vi "Read_Write_ADAM_setup.vi"(3 "Mode":T1(ring)) -> ()   [LabVIEW 2012]
uses:
  ADAM Client/Sub VIs/ADAM Controls/Channel_State.ctl
  Anemometry/Anemometry Sub Vis/Globals/Constants_global.vi
  Anemometry/Anemometry Sub Vis/Globals/Gas_management_global.vi
  Exp conditions/EnFlo_Tun_Setup_global.vi
  ADAM_Global.vi
  Channel_Description_Global.vi
panel:
  out "Setup Filename":string
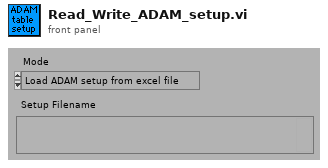
[diagram p1: front panel]
types:
  T1 = enum16{"Load ADAM setup from excel file", "Save ADAM setup to excel file"}
  T2 = typedef "Channel_State.ctl" = enum16{"On", "Off", "Always On", "Always Off"}
  T3 = typedef "Ch_description_ADAM.ctl" = cluster{"Ch Name":string, "Type":T4, "Function":T5, "Ch State":T2, "Calibration type":T6, "A":dbl, "B":dbl, "C":dbl, "D":dbl, "Comments":string, "Address":T7, "String":string, "Duty":u16}
  T4 = typedef "Module_type_ADAM.ctl" = string
  T5 = typedef "Function_ADAM.ctl" = enum16{"Analogue Input", "Digital Input", "Event counter", "Event rate", "Analogue Output", "Digital Output", "Relay Output"}
  T6 = typedef "Calib_type_ADAM.ctl" = enum16{"Raw", "Bx + A", "Cx^2 + Bx + A", "Dx^3 + Cx^2 + Bx + A", "In Band", "Hi-Tec Q", "Hi-Tec M_dot", "Text"}
  T7 = typedef "Address.ctl" = cluster{"Main":i32, "Ch.":i32, "Sub":i32, "Port Name":string}
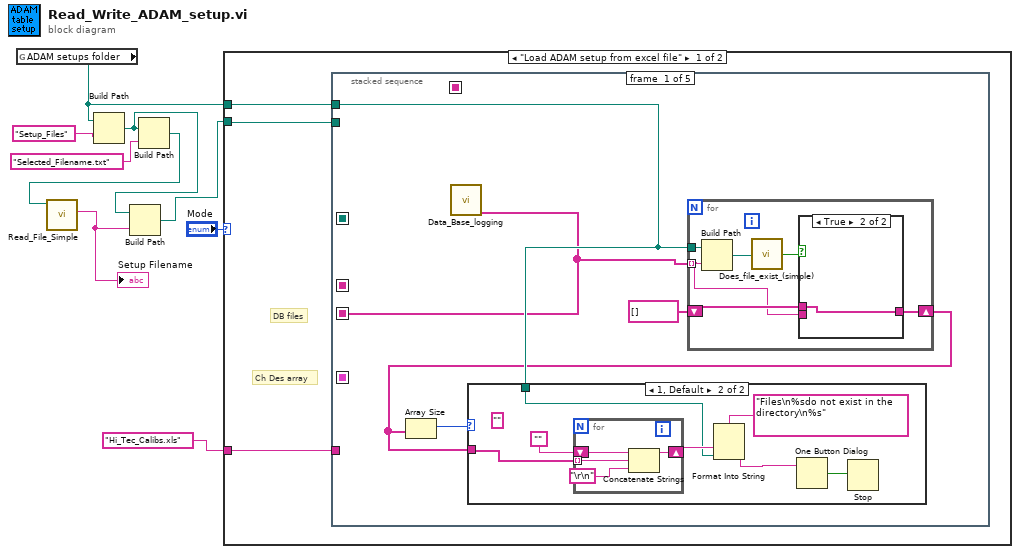
[diagram p0: block diagram]
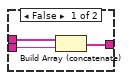
[diagram p3: hidden frame]
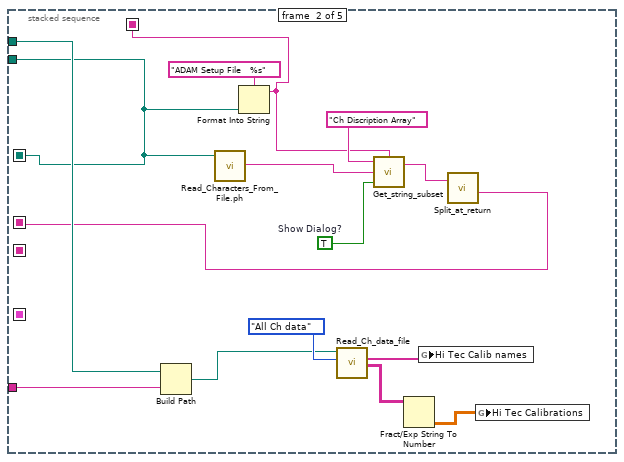
[diagram p4: hidden frame]
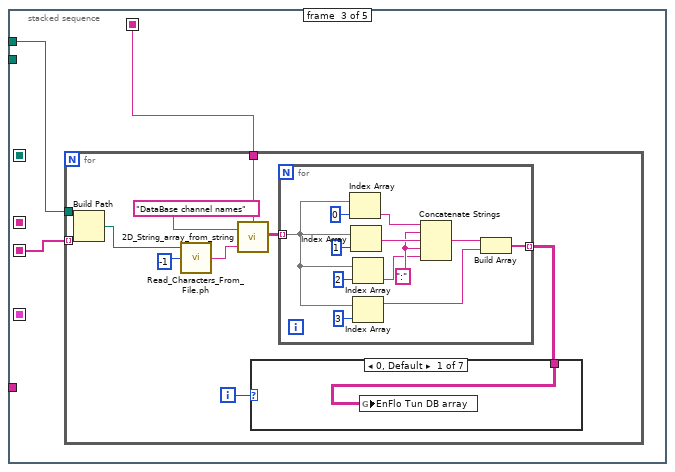
[diagram p5: hidden frame]
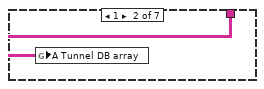
[diagram p6: hidden frame]
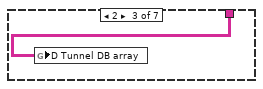
[diagram p7: hidden frame]
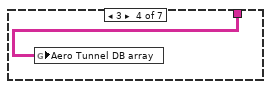
[diagram p8: hidden frame]
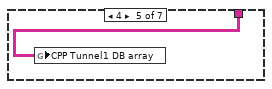
[diagram p9: hidden frame]
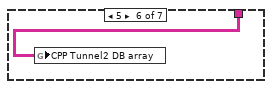
[diagram p10: hidden frame]
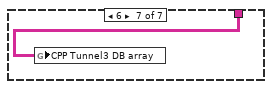
[diagram p11: hidden frame]
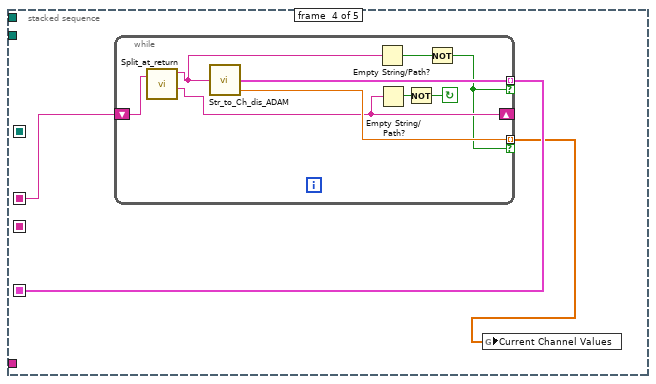
[diagram p12: hidden frame]
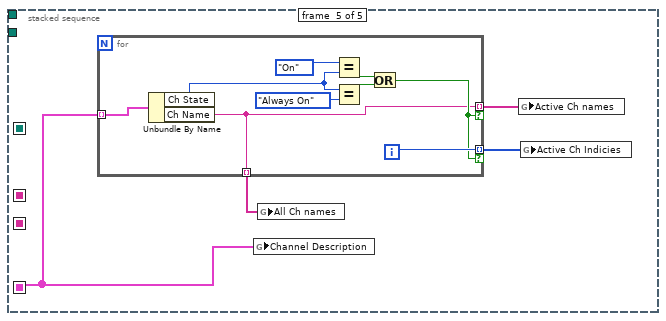
[diagram p13: hidden frame]
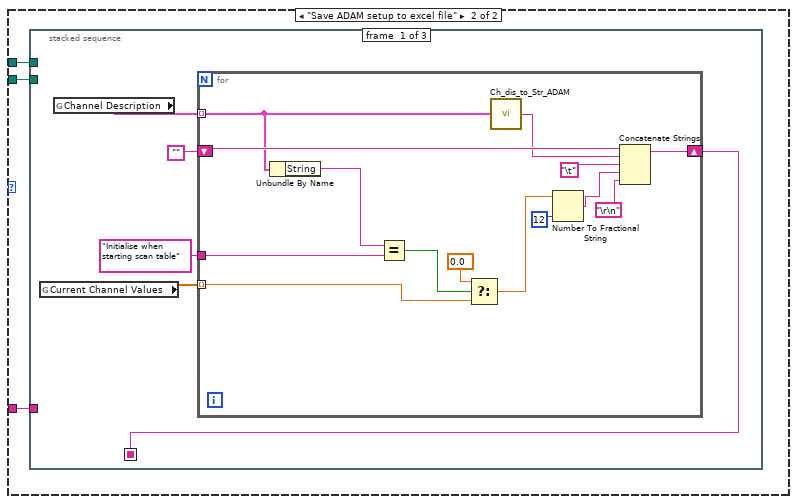
[diagram p14: hidden frame]
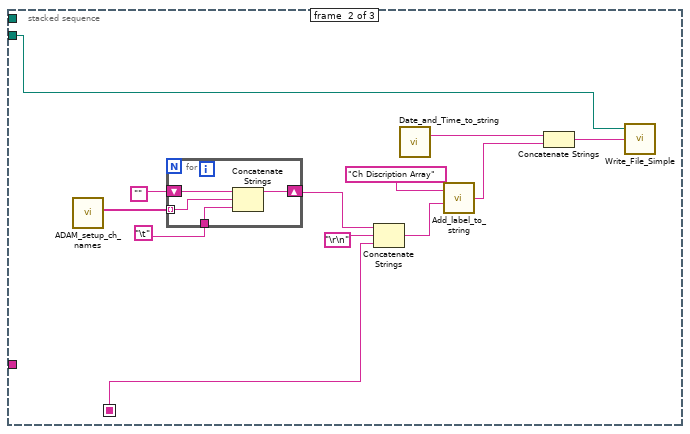
[diagram p15: hidden frame]
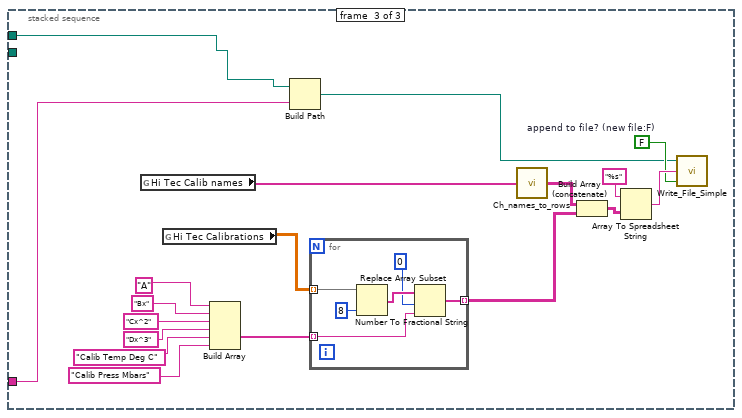
[diagram p16: hidden frame]
diagram:
  n1 = global read "Constants_global.vi" "ADAM setups folder"() -> (w8:path)
  n2 = Build Path(base path=w8, name or relative path="Setup_Files") -> (appended path=w4:path)
  n3 = Build Path(base path=w4, name or relative path="Selected_Filename.txt" ("Substring")) -> (appended path=w5:path)
  n4 = call "Read_File_Simple.vi"("Filename"=w5) -> ("string"=w3:string)  [unwired: 2 in, 7 out]
  "Setup Filename" <- w3
  n5 = Build Path(base path=w4, name or relative path=w3) -> (appended path=w2:path)
  n6 = case shown="\"Load ADAM setup from excel file\"" "Mode" {
    tunnel: w2 -> [w12 w113]
    tunnel: w8 -> [w11 w112]
    tunnel: "Hi_Tec_Calibs.xls" ("name or relative path") -> [w10 w111]
    frame "Load ADAM setup from excel file" {
      # "DB files"
      # "Ch Des array"
      n7 = stacked-sequence {
        seq-local: [_ w42 _ _ _] -> [_ _ _ w88 _]
        seq-local: [_ _ _ w87 _] -> [_ _ _ _ w101]
        seq-local: [_ w40 _ _ _] -> [_ _ _ _ _]
        seq-local: [w13 _ _ _ _] -> [_ _ w55 _ _]
        seq-local: [_ w39 _ _ _] -> [_ _ w54 _ _]
        tunnel: w12 -> [_ w40 _ _ _]
        tunnel: w11 -> [w15 w47 w56 _ _]
        tunnel: w10 -> [_ w44 _ _ _]
        frame #0 {
          n8 = call "Data_Base_logging.vi"() -> ("DB Setup files"=w13:string[])  [unwired: 4 out]
          n9 = for {
            tunnel: w13 -> [w30] mode=indexing
            tunnel: w15 -> [w34]
            shift-right: [w29] -> w14
            shift-left: string[] [] -> [w31]
            n10 = Build Path(base path=w34, name or relative path=w30) -> (appended path=w33:path)
            n11 = call "Does_file_exist_(simple).vi"("Pathname"=w33) -> ("exists?"=w32:bool)
            n12 = case shown="True" w32 {
              tunnel: w31 -> [w37 w38]
              tunnel: w30 -> [w36 _]
              tunnel: [w35 w38] -> w29
              frame False {
                n13 = Build Array (concatenate)(w37, w36) -> (w35:string[])
              }
              frame True {
              }
            }
          }
          n14 = Array Size(array=w14) -> (size(s)=w16:i32)
          n15 = case shown="1, Default" w16 {
            tunnel: w15 -> [_ w21]
            tunnel: w14 -> [_ w23]
            frame 0 {
            }
            frame 1, Default {
              (unwired) ""
              n16 = for {
                shift-right: [w25] -> w22
                shift-left: "" -> [w28]
                tunnel: w23 -> [w26] mode=indexing
                n17 = Concatenate Strings(w28, w26, "\r\n") -> (w25:string)
              }
              n18 = Format Into String(format string="Files\n%sdo not exist in the directory\n%s" ("Format String"), w22, w21) -> (resulting string=w19:string)  [unwired: 2 in, 1 out]
              n19 = One Button Dialog(message=w19) -> (true=w18:bool)  [unwired: 1 out]
              n20 = Stop(stop? (T)=w18) -> ()
            }
          }
        }
        frame #1 {
          w48 = TRUE  # Show Dialog?
          n21 = Build Path(base path=w47, name or relative path=w44) -> (appended path=w46:path)
          n22 = call "Read_Characters_From_File.ph.vi"("file path (dialog if empty)"=w40) -> ("character string"=w45:string)  [unwired: 1 in, 7 out]
          n23 = Format Into String(format string="ADAM Setup File   %s", w40) -> (resulting string=w39:string)  [unwired: 2 in, 1 out]
          n24 = call "Read_Ch_data_file.vi"("Output"=enum16{"All Ch data", "The last few rows"}."All Ch data", "Filename"=w46) -> ("Channel Values"=w50:string[][], "Merged Channels"=w51:string[])  [unwired: 3 in, 3 out]
          n25 = call "Get_string_subset.vi"("String Name"=w39, "Show Dialog?"=w48, "String to split"=w45, "File Label"="Ch Discription Array") -> ("Output string"=w43:string)  [unwired: 1 out]
          n26 = Fract/Exp String To Number(string=w50) -> (number=w49:dbl[][])  [unwired: 4 out]
          n27 = global write "Gas_management_global.vi" "Hi Tec Calib names"(w51) -> ()
          n28 = call "Split_at_return.vi"("String"=w43) -> ("after substring"=w42:string)  [unwired: 1 in, 3 out]
          n29 = global write "Gas_management_global.vi" "Hi Tec Calibrations"(w49) -> ()
        }
        frame #2 {
          n30 = for {
            tunnel: w56 -> [w60]
            tunnel: w55 -> [w59] mode=indexing
            tunnel: w54 -> [w57]
            i -> [w62]
            n31 = Build Path(base path=w60, name or relative path=w59) -> (appended path=w58:path)
            n32 = call "Read_Characters_From_File.ph.vi"("file path (dialog if empty)"=w58, "number of characters (all:-1)"=-1) -> ("character string"=w63:string)  [unwired: 7 out]
            n33 = call "2D_String_array_from_string.vi"("String Name"=w57, "Input string"=w63, "Array title"="DataBase channel names") -> ("2D data array"=w64:string[][])
            n34 = for {
              tunnel: w64 -> [w77] mode=indexing
              tunnel: [w75] -> w61 mode=indexing
              w80 = ":"
              n35 = Index Array(array=w77, index=0) -> (element=w82:string)
              n36 = Index Array(array=w77, index=1) -> (element=w81:string)
              n37 = Index Array(array=w77, index=2) -> (element=w79:string)
              n38 = Index Array(array=w77, index=3) -> (element=w76:string)
              n39 = Concatenate Strings(w82, w80, w81, w80, w79) -> (w74:string)
              n40 = Build Array(w74, w76) -> (w75:string[])
            }
            n41 = case shown="0, Default" w62 {
              tunnel: w61 -> [w67 w68 w69 w70 w71 w72 w73]
              frame 0, Default {
                n42 = global write "EnFlo_Tun_Setup_global.vi" "EnFlo Tun DB array"(w67) -> ()
              }
              frame 1 {
                n43 = global write "EnFlo_Tun_Setup_global.vi" "A Tunnel DB array"(w68) -> ()
              }
              frame 2 {
                n44 = global write "EnFlo_Tun_Setup_global.vi" "D Tunnel DB array"(w69) -> ()
              }
              frame 3 {
                n45 = global write "EnFlo_Tun_Setup_global.vi" "Aero Tunnel DB array"(w70) -> ()
              }
              frame 4 {
                n46 = global write "EnFlo_Tun_Setup_global.vi" "CPP Tunnel1 DB array"(w71) -> ()
              }
              frame 5 {
                n47 = global write "EnFlo_Tun_Setup_global.vi" "CPP Tunnel2 DB array"(w72) -> ()
              }
              frame 6 {
                n48 = global write "EnFlo_Tun_Setup_global.vi" "CPP Tunnel3 DB array"(w73) -> ()
              }
            }
          }
        }
        frame #3 {
          n49 = while {
            tunnel: [w94] -> w86 mode=indexing if=w89
            tunnel: [w95] -> w87 mode=indexing if=w89
            shift-left: w88 -> [w92]
            shift-right: [w93] -> _
            stop <- w96 continue-if-true
            n50 = call "Split_at_return.vi"("String"=w92) -> ("before substring"=w91:string, "after substring"=w93:string)  [unwired: 1 in, 2 out]
            n51 = call "Str_to_Ch_dis_ADAM.vi"("String Row"=w91) -> ("Value"=w94:dbl, "Ch Description"=w95:T3)  [unwired: 1 in, 2 out]
            n52 = Empty String/Path?(string/path=w91) -> (empty?=w90:bool)
            n53 = Empty String/Path?(string/path=w93) -> (empty?=w97:bool)
            n54 = Not(x=w97) -> (.not. x?=w96:bool)
            n55 = Not(x=w90) -> (.not. x?=w89:bool)
          }
          n56 = global write "ADAM_Global.vi" "Current Channel Values"(w86) -> ()
        }
        frame #4 {
          n57 = for {
            tunnel: w101 -> [w105] mode=indexing
            tunnel: [w102] -> w100 mode=indexing if=w103
            tunnel: [w104] -> w99 mode=indexing if=w103
            tunnel: [w102] -> w98 mode=indexing
            i -> [w104]
            n58 = Unbundle By Name(w105) -> ("Ch State"=w106:T2, "Ch Name"=w102:string)
            n59 = Equal?(x=Channel_State."On" ("Channel State"), y=w106) -> (x = y?=w108:bool)
            n60 = Equal?(x=w106, y=Channel_State."Always On" ("Channel State")) -> (x = y?=w107:bool)
            n61 = Or(x=w108, y=w107) -> (x .or. y?=w103:bool)
          }
          n62 = global write "Channel_Description_Global.vi" "Channel Description"(w101) -> ()
          n63 = global write "ADAM_Global.vi" "All Ch names"(w98) -> ()
          n64 = global write "ADAM_Global.vi" "Active Ch names"(w100) -> ()
          n65 = global write "ADAM_Global.vi" "Active Ch Indicies"(w99) -> ()
        }
      }
    }
    frame "Save ADAM setup to excel file" {
      n66 = stacked-sequence {
        seq-local: [w117 _ _] -> [_ w137 _]
        tunnel: w113 -> [_ w134 _]
        tunnel: w112 -> [_ _ w158]
        tunnel: w111 -> [_ _ w157]
        frame #0 {
          n67 = global read "ADAM_Global.vi" "Current Channel Values"() -> (w116:dbl[])
          n68 = global read "Channel_Description_Global.vi" "Channel Description"() -> (w114:T3[])
          n69 = for {
            shift-right: [w119] -> w117
            shift-left: "" -> [w132]
            tunnel: w114 -> [w131] mode=indexing
            tunnel: w116 -> [w130] mode=indexing
            tunnel: "Initialise when starting scan table" ("y") -> [w129]
            n70 = Unbundle By Name(w131) -> ("String"=w122:string)
            n71 = Equal?(x=w122, y=w129) -> (x = y?=w121:bool)
            n72 = Select(t=0.0, s=w121, f=w130) -> (s? t:f=w123:dbl)
            n73 = call "Ch_dis_to_Str_ADAM.vi"("Ch Description"=w131) -> ("String Row"=w128:string)  [unwired: 4 out]
            n74 = Number To Fractional String(number=w123, precision (6)=i16 12) -> (F-format string=w124:string)  [unwired: 2 out]
            n75 = Concatenate Strings(w132, w128, "\t", w124, "\r\n") -> (w119:string)
          }
        }
        frame #1 {
          n76 = call "ADAM_setup_ch_names.vi"() -> ("Ch Names"=w136:string[])  [unwired: 1 out]
          n77 = for {
            shift-right: [w145] -> w135
            shift-left: "" -> [w148]
            tunnel: "\t" -> [w146]
            tunnel: w136 -> [w147] mode=indexing
            n78 = Concatenate Strings(w148, w147, w146) -> (w145:string)
          }
          n79 = Concatenate Strings(w135, "\r\n", w137) -> (w143:string)
          n80 = call "Date_and_Time_to_string.vi"() -> ("Date and time (spreadsheet)"=w142:string)
          n81 = call "Add_label_to_string.vi"("String to write"=w143, "File Label"="Ch Discription Array") -> ("Output string"=w141:string)
          n82 = Concatenate Strings(w142, w141) -> (w133:string)
          n83 = call "Write_File_Simple.vi"("character string"=w133, "file path"=w134) -> ()  [unwired: 1 in, 2 out]
        }
        frame #2 {
          w152 = FALSE  # append to file? (new file:F)
          n84 = global read "Gas_management_global.vi" "Hi Tec Calib names"() -> (w150:string[])
          n85 = global read "Gas_management_global.vi" "Hi Tec Calibrations"() -> (w166:dbl[][])
          n86 = Build Array("A", "Bx", "Cx^2", "Dx^3", "Calib Temp Deg C", "Calib Press Mbars") -> (w159:string[])
          n87 = Build Path(base path=w158, name or relative path=w157) -> (appended path=w151:path)
          n88 = for {
            tunnel: w166 -> [w172] mode=indexing
            tunnel: [w169] -> w149 mode=indexing
            tunnel: w159 -> [w167] mode=indexing
            n89 = Number To Fractional String(number=w172, precision (6)=i16 8) -> (F-format string=w170:string[])  [unwired: 2 out]
            n90 = Replace Array Subset(array=w170, new element=w167, index=0) -> (w169:string[])
          }
          n91 = call "Ch_names_to_rows.vi"("Channel Names"=w150) -> ("3 Row names"=w156:string[][])
          n92 = Build Array (concatenate)(w156, w149) -> (w154:string[][])
          n93 = Array To Spreadsheet String(array=w154, 3:"%s" ("format string")) -> (spreadsheet string=w153:string)  [unwired: 1 out]
          n94 = call "Write_File_Simple.vi"("append to file? (new file:F)"=w152, "character string"=w153, "file path"=w151) -> ()  [unwired: 2 out]
        }
      }
    }
  }
